vi "CRYSet Harmonics List Editor Front Panel.vi"(11 "Vi Ref":refnum<vi>) -> ()   [LabVIEW 2013]
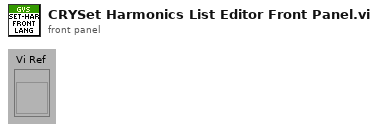
[diagram p1: front panel]
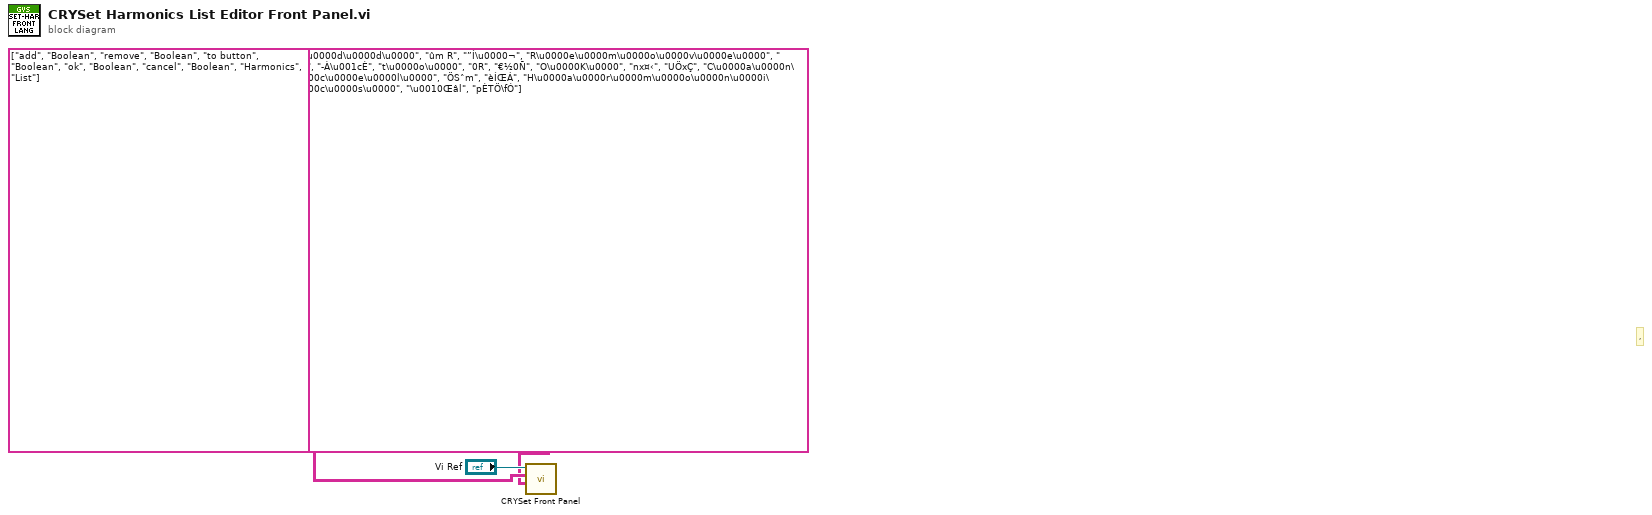
[diagram p0: block diagram]
diagram:
  # ","
  # "Caption, Tab Page, Multilist Header, Button 4"
  # "Control Type"
  # "Control Name and Tab"
  n1 = call "CRYSet Front Panel.vi"("Caption(Boolean Text)"=string[][] [["A\u0000d\u0000d\u0000", "ûm R", "”Í\u0000¬"], ["R\u0000e\u0000m\u0000o\u0000v\u0000e\u0000", " Rd–", "­À\u001cÈ"], ["t\u0000o\u0000", "0R", "€½0Ñ"], ["O\u0000K\u0000", "nx¤‹", "UÖxÇ"], ["C\u0000a\u0000n\u0000c\u0000e\u0000l\u0000", "ÖSˆm", "èÍŒÁ"], ["H\u0000a\u0000r\u0000m\u0000o\u0000n\u0000i\u0000c\u0000s\u0000", "\u0010Œâl", "pÈTÖ\fÓ"]], "Control ID and Type(Label Name, Type)"=string[][] [["add", "Boolean"], ["remove", "Boolean"], ["to button", "Boolean"], ["ok", "Boolean"], ["cancel", "Boolean"], ["Harmonics", "List"]], "Vi Ref"="Vi Ref") -> ()  [unwired: 9 in]
